vi "Set Channel to External Source.vi"(5 "return state (tristate)":T1=90 items=["Tristate"=90, "Previous digital state"=91], 7 "action":u32(ring)=92 items=["Connect"=92, "Disconnect"=93], 8 "error in (no error)":errorcluster, 10 "Pins for external Source":string[](array[string]), 11 "Semiconductor Module Context":T2) -> (0 "error out":errorcluster)   [LabVIEW 2013]
uses:
  <vilib>/NI_TestStand_SemiconductorModule/NI_TestStand_Semiconductor_Module.lvlibp/PinMap/General/SemiconductorModuleContext.ctl
  <instrlib>/niHSDIO/niHSDIO.llb/niHSDIO_ctl stPMU Disable Return State.ctl
  <instrlib>/niHSDIO/niHSDIO.llb/niHSDIO_ctl stPMU Connector Values.ctl
  <vilib>/NI_TestStand_SemiconductorModule/NI_TestStand_Semiconductor_Module.lvlibp/PinMap/HSDIO/PinsToNIHSDIOSessions.vi
  <vilib>/NI_TestStand_SemiconductorModule/NI_TestStand_Semiconductor_Module.lvlibp
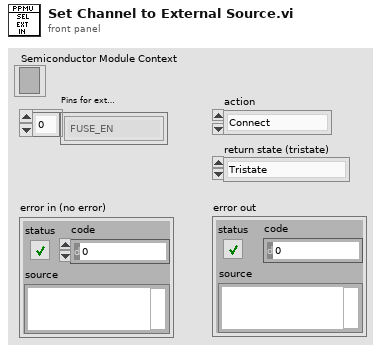
[diagram p1: front panel]
types:
  T1 = typedef "niHSDIO_ctl stPMU Disable Return State.ctl" = u32
  T2 = typedef "NI_TestStand_Semiconductor_Module.lvlibp/SemiconductorModuleContext.ctl" = refnum<k7>
  T3 = typedef "niHSDIO_ctl stPMU Connector Values.ctl" = u32
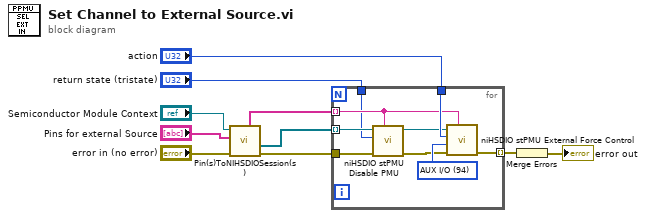
[diagram p0: block diagram]
diagram:
  n1 = call-poly <vilib>:"Pin(s)ToNIHSDIOSession(s).vi"("error in (no error)"="error in (no error)", "Pins"="Pins for external Source", "Semiconductor Module Context"="Semiconductor Module Context") -> ("error out"=w10:errorcluster, "Generation Sessions"=w9:refnum<k15>[], "Channel Lists"=w8:string[])  [unwired: 3 in, 3 out]
  n2 = for {
    tunnel: w10 -> [w16]
    tunnel: w9 -> [w12] mode=indexing
    tunnel: w8 -> [w13] mode=indexing
    tunnel: [w19] -> w5 mode=indexing
    tunnel: "action" -> [w17]
    tunnel: "return state (tristate)" -> [w11]
    w18 = T3 94 items=["AUX I/O"=94, "Remote Sense"=95] ("connector")
    n3 = call <instrlib>:"niHSDIO stPMU Disable PMU.vi"("channel list"=w13, "error in (no error)"=w16, "return state (tristate)"=w11, "instrument handle"=w12) -> ("error out"=w15:errorcluster, "instrument handle out"=w14:refnum<k15>)  [unwired: 6 in]
    n4 = call <instrlib>:"niHSDIO stPMU External Force Control.vi"("channel list"=w13, "error in (no error)"=w15, "connector"=w18, "action"=w17, "instrument handle"=w14) -> ("error out"=w19:errorcluster)  [unwired: 5 in, 1 out]
  }
  n5 = Merge Errors(w5) -> (→"error out":errorcluster)
